vi "Update SDI.vi"(8 "error in":errorcluster, 10 "SDI value":u8 format="%02b", 11 "32-bit Word in":refnum<class "32-bit Word.lvclass">) -> (0 "error out":errorcluster, 3 "32-bit Word out":refnum<class "32-bit Word.lvclass">)   [LabVIEW 2020, in "32-bit Word.lvclass"]
uses:
  32-bit Word.lvclass
  32-bit Word.lvclass/32-bit Word.ctl
  5f5aa9c9-dfb1-442a-a7d8-deed5716d765.vi
  Read 32-Bit Word.vi
  Read SDI Start Index.vi
  Read SDI Size.vi
  Write 32-Bit Word.vi
  Write SDI Value.vi
  5f5aa9c9-dfb1-442a-a7d8-deed5716d765.vi/9935dc85-f143-411c-b80b-16b6c96eb14a.vi
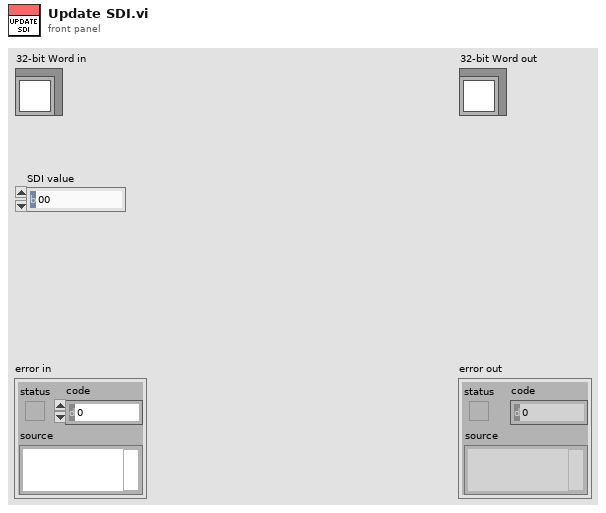
[diagram p1: front panel]
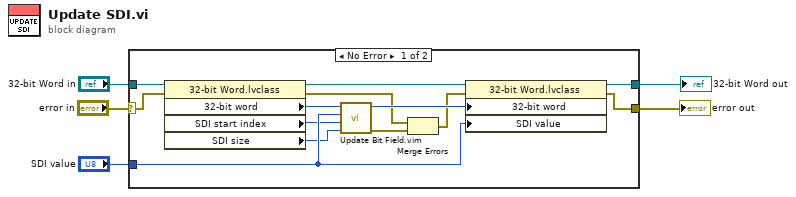
[diagram p0: block diagram]
diagram:
  n1 = case shown="No Error" "error in" {
    selector: "error in" -> [w15 w20]
    tunnel: [w14 w20] -> w4
    tunnel: [w16 w19] -> w2
    tunnel: "32-bit Word in" -> [w18 w19]
    tunnel: "SDI value" -> [w11 _]
    frame No Error {
      n2 = property class="32-bit Word.lvclass"(reference=w18, error in=w15) -> (reference out=w17:refnum<class "32-bit Word.lvclass">, error out=w7:errorcluster, "32-bit word"=w13:u32, "SDI start index"=w10:i32, "SDI size"=w9:i32)
      n3 = call "Update Bit Field.vim"("bit field size"=w9, "bit field start index"=w10, "value"=w11, "word in"=w13) -> ("error out"=w8:errorcluster, "word out"=w12:u32)  [unwired: 6 in]
      n4 = Merge Errors(w7, w8) -> (w6:errorcluster)
      n5 = property class="32-bit Word.lvclass"(reference=w17, error in=w6, "32-bit word"=w12, "SDI value"=w11) -> (reference out=w16:refnum<class "32-bit Word.lvclass">, error out=w14:errorcluster)
    }
    frame Error {
    }
  }
  "error out" <- w4
  "32-bit Word out" <- w2
